vi "Byte Buffer.Read (1D U16).vi"(8 "error in (no error)":errorcluster, 9 "count":i64, 10 "buffer offset":u64, 11 "Byte Buffer in":refnum<class "Byte Buffer.lvclass">) -> (0 "error out":errorcluster, 1 "value":u16[](array[numeric]), 2 "new buffer offset":u64, 3 "Byte Buffer out":refnum<class "Byte Buffer.lvclass">)   [LabVIEW 2016, in "VeriStand Data.lvlib" / "Byte Buffer.lvclass"]
doc: "Reads <B>count</B> elements of data from the provided <B>Byte Buffer</B> at location <B>buffer offset</B> in the format of the data type specified."
uses:
  Byte Buffer.lvclass
  Typedefs/Typedefs.Data Types.ctl
  Byte Buffer.lvclass/Byte Buffer.ctl
  Byte Buffer.Subset.Get.vi
  Utilities/Utilities.Sizeof.Array.vi
  Utilities/Utilities.Buffer.String.vi
  Memory Management/Memory Management.MoveByteBlock.Write (String).vi
  Utilities/Utilities.Sizeof.Scalar.vi
  Memory Management/Memory Management.Handle Return.vi
  VeriStand Data.lvlib
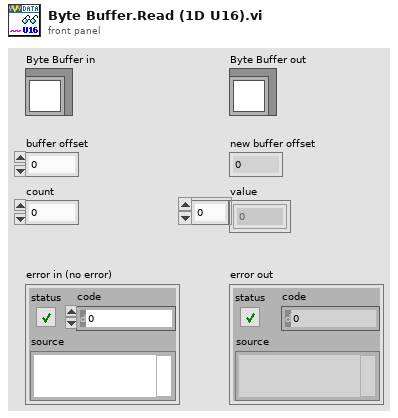
[diagram p1: front panel]
types:
  T1 = typedef "VeriStand Data.lvlib/Typedefs.Data Types.ctl" = enum16{"Boolean", "Single", "Double", "I8", "I16", "I32", "I64", "U8", "U16", "U32", "U64"}
  T2 = enum16{"big-endian, network order", "native, host order", "little-endian"}
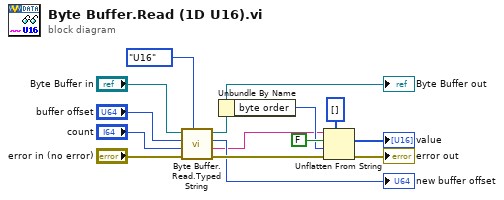
[diagram p0: block diagram]
diagram:
  n1 = call "Byte Buffer.Read.Typed String.vi"("data type"=Typedefs.Data_Types."U16", "error in (no error)"="error in (no error)", "count"="count", "buffer offset"="buffer offset", "Byte Buffer in"="Byte Buffer in") -> ("error out"=w9:errorcluster, "string"=w1:string, "new buffer offset"=→"new buffer offset":u64, "Byte Buffer out"=w6:refnum<class "Byte Buffer.lvclass">)  [unwired: 3 in]
  "Byte Buffer out" <- w6
  n2 = Unbundle By Name(w6) -> ("byte order"=w5:T2)
  n3 = Unflatten From String(type=u16[] [], binary string=w1, data includes array or string size? (T)=FALSE, byte order (0:big-endian, network order)=w5, error in (no error)=w9) -> (value=→"value":u16[], error out=→"error out":errorcluster)  [unwired: 1 out]
